vi "Scanning Motion One Direction for Y Multiple Readings per Point.vi"() -> ()   [LabVIEW 2021]
uses:
  <vilib>/Utility/file.llb/Write Delimited Spreadsheet (DBL).vi
  MID-main/Marlin Instrument Driver/Marlin Instrument Driver.lvlib
  <instrlib>/Siglent SDS 1000 2000 Series/Siglent SDS 1000 2000 Series.lvlib
panel:
  in  "Samples per pt":dbl=10.0
  in  "VISA resource name o-scope":refnum<visa-resource-name>="USB0::0xF4ED::0xEE3A::SDS1EDED5R2476::INSTR"
  in  "Measurement (0: Vpp)":u16(ring) items=["Vpp", "Vmax", "Vmin", "Vamp", "Vtop", "Vbase", "Vavg", "Mean", "Vrms", "Crms", "FOV", "FPRE", "ROV", "RPRE", "Period", "Freq", "+Wid", "-Wid", "Rise Time", "Fall Time", "Bwid", "+Duty", "-Duty"]
  in  "Source (1: Channel 1)":u16(ring)=1 items=["Channel 1"=1, "Channel 2"=2, "Channel 3"=3, "Channel 4"=4]
  in  "file path (dialog if empty)":path=path "C:/Users/scoughen/Documents/Printer Controll/Coughenour Programs/Scan Data/SimpleTransducer500kHzHighRes10SampleAvg0SecDelay7mmOffsetFromTransducerNewAmp.csv"
  in  "T":dbl
  in  "y Flag":string="Negative"
  in  "x Flag":string="Negative"
  in  "linearF":dbl=1000.0
  in  "E":dbl
  in  "rapidF":dbl=3000.0
  in  "zRes":dbl=0.5
  in  "yRes":dbl=1.0
  in  "xRes":dbl=0.5
  in  "zSize":dbl=80.0
  in  "ySize":dbl=10.0
  in  "xSize":dbl=50.0
  in  "zInit":dbl=155.0
  in  "yInit":dbl=168.0
  in  "xInit":dbl=115.0
  out "error out":errorcluster
  in  "error in (no error)":errorcluster
  in  "VISA resource name":refnum<visa-resource-name>="COM5"
  # "All Units in mm"
  # "Initial Position"
  # "Scan Size"
  # "Scan Resolution"
  # "Extrusion"
  # "Feed Rate"
  # "Read Delay (s)"
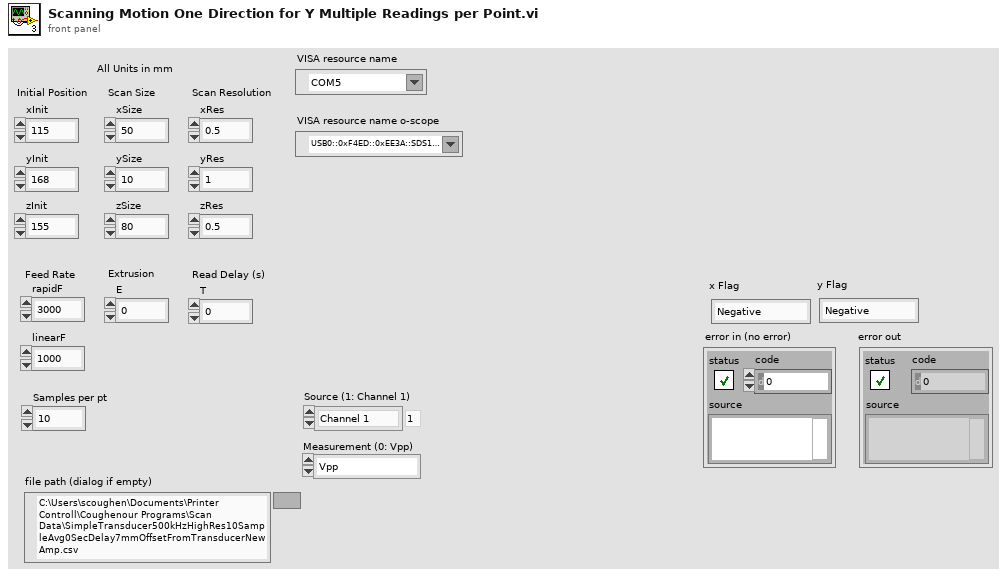
[diagram p1: front panel]
types:
  T1 = cluster{"E":dbl, "rapidF":dbl, "xInit":dbl, "yInit":dbl, "zInit":dbl}
  T2 = cluster{"E":dbl, "linearF":dbl, dbl, "yInit":dbl, "zInit":dbl}
  T3 = cluster{"E":dbl, "linearF":dbl, "xInit":dbl, dbl, "zInit":dbl}
  T4 = cluster{"E":dbl, "linearF":dbl, dbl, "zInit":dbl, "yInit":dbl}
  T5 = cluster{"E":dbl, "linearF":dbl, "xInit":dbl, "yInit":dbl, dbl}
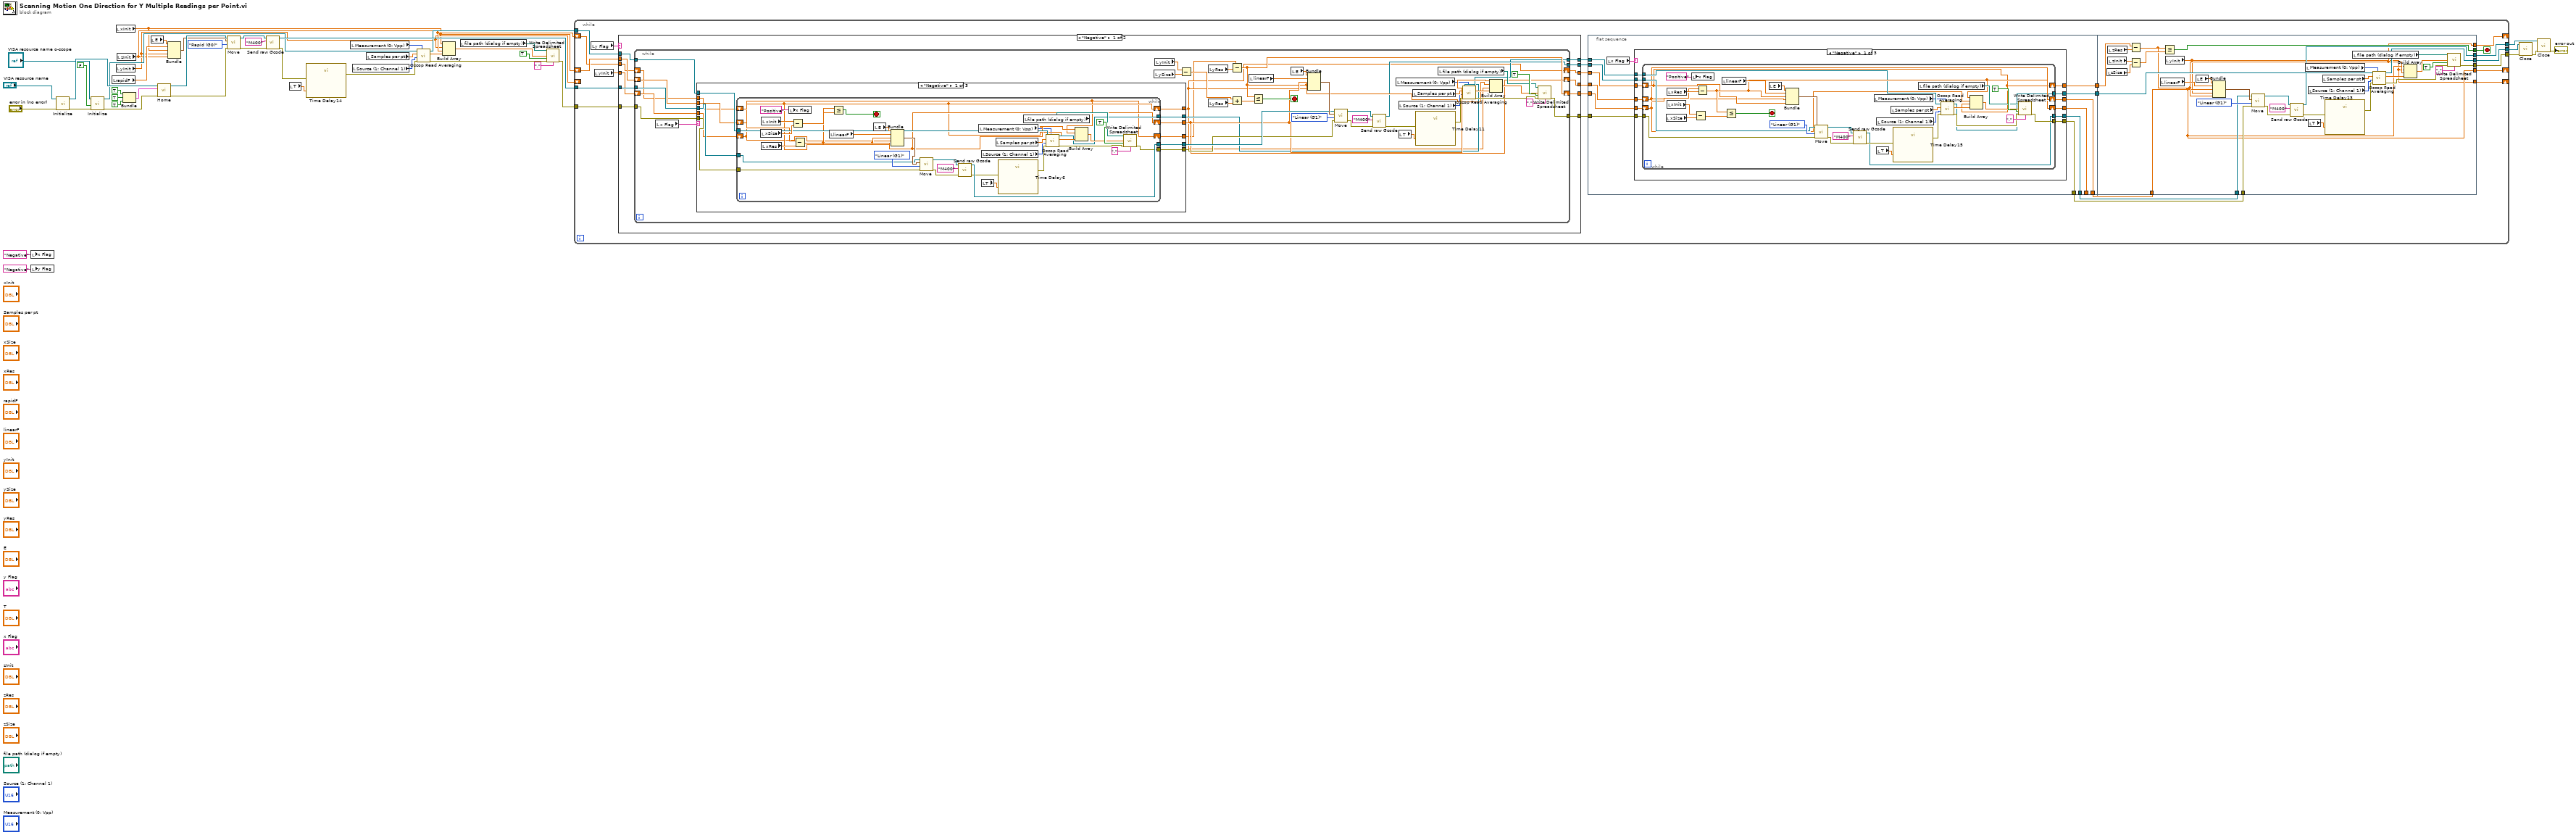
[diagram p0: block diagram]
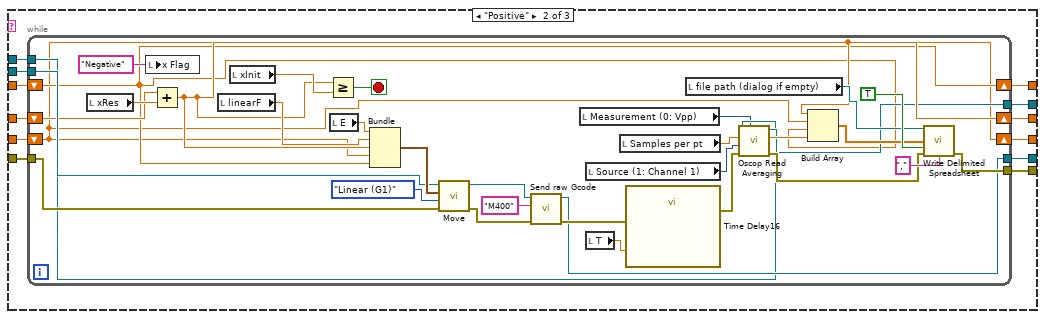
[diagram p2: hidden frame]
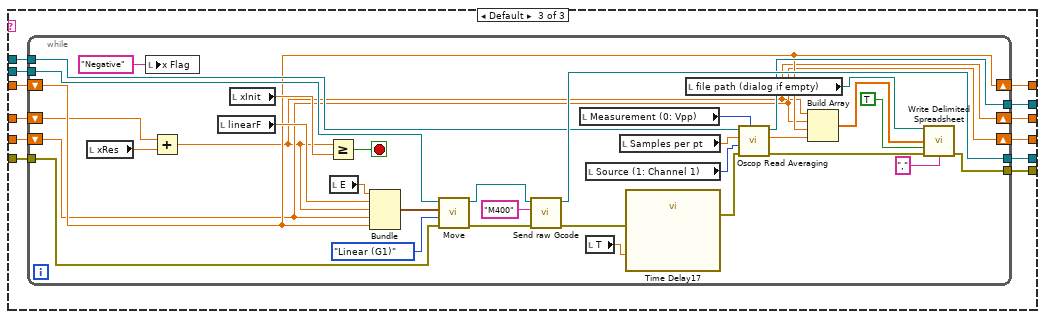
[diagram p3: hidden frame]
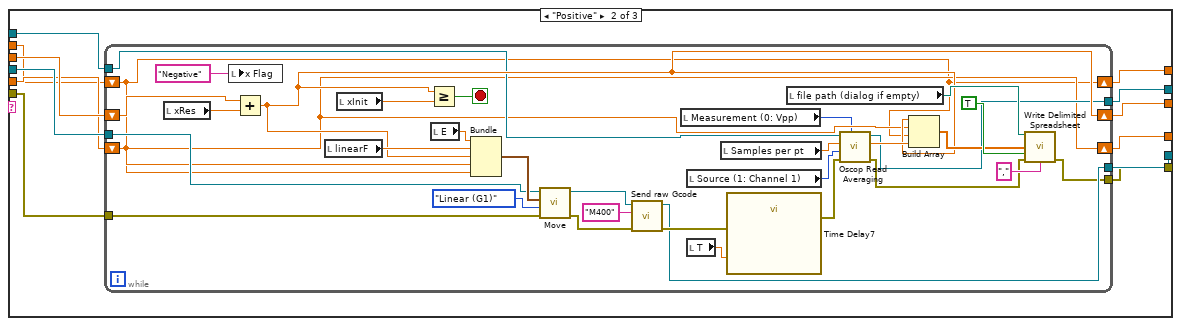
[diagram p4: hidden frame]
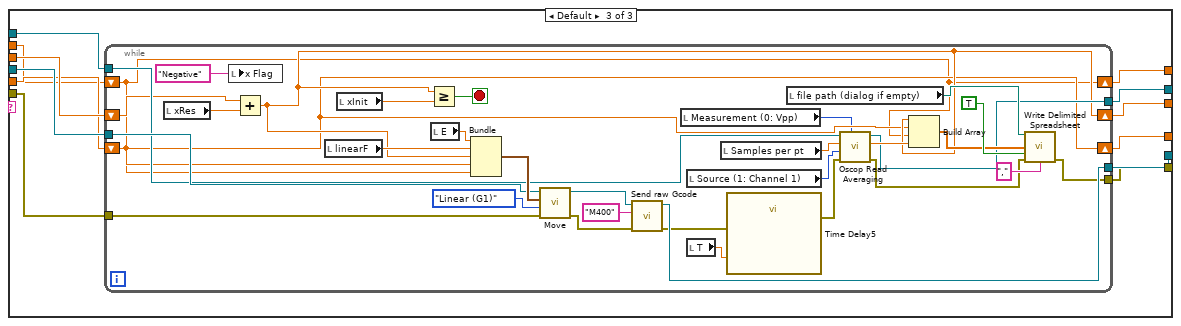
[diagram p5: hidden frame]
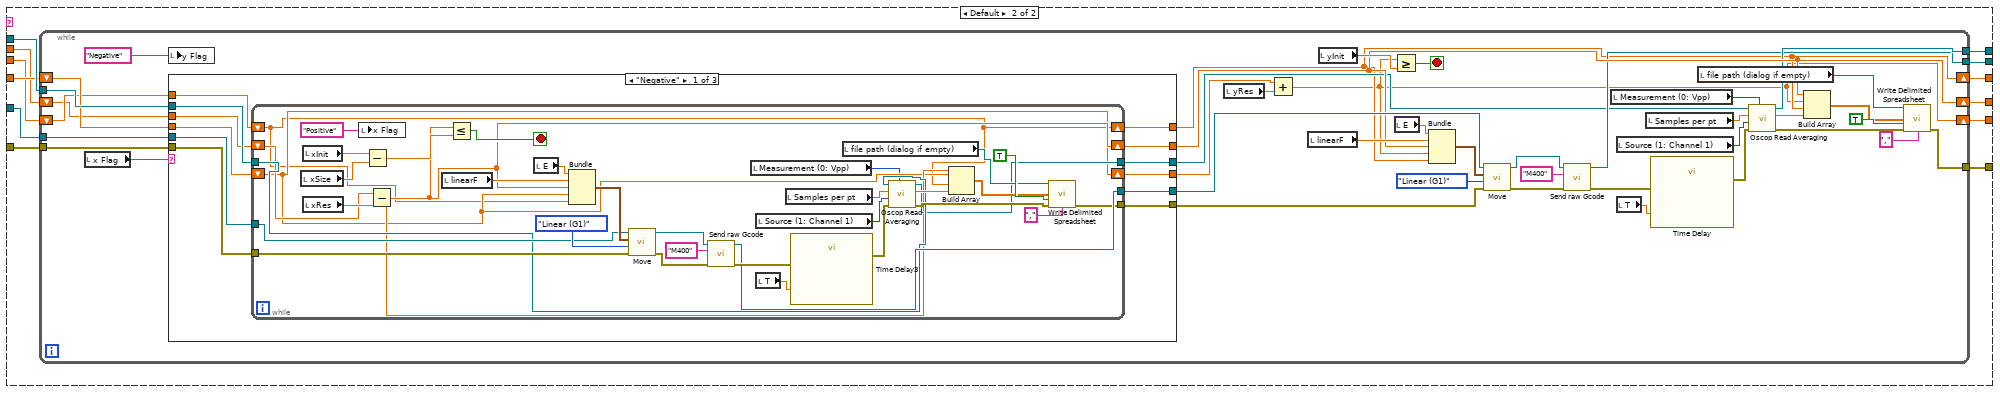
[diagram p6: hidden frame]
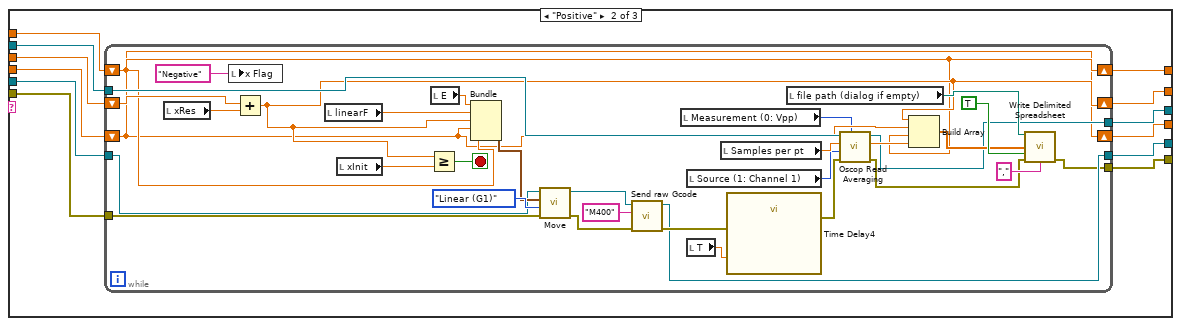
[diagram p7: hidden frame]
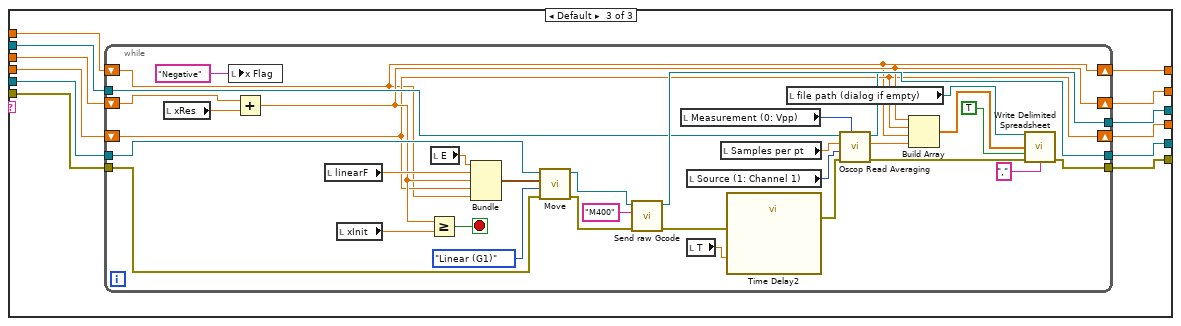
[diagram p8: hidden frame]
diagram:
  n1 = local write "x Flag"("Negative" ("x Flag")) -> ()
  n2 = local write "y Flag"("Negative" ("y Flag")) -> ()
  n3 = call <instrlib>:"Initialize.vi"("error in (no error)"="error in (no error)", "VISA resource name"="VISA resource name") -> ("error out"=w23:errorcluster, "VISA resource name out"=w43:refnum<visa-resource-name>)  [unwired: 8 in]
  n4 = call <instrlib>:"Initialize.vi"("error in (no error)"=w23, "Reset (True)"=FALSE, "VISA resource name"="VISA resource name o-scope") -> ("error out"=w22:errorcluster, "VISA resource name out"=w11:refnum<visa-resource-name>)  [unwired: 7 in]
  n5 = local read "rapidF"() -> (w33:dbl)
  n6 = local read "xInit"() -> (w6:dbl)
  n7 = local read "yInit"() -> (w7:dbl)
  n8 = local read "zInit"() -> (w8:dbl)
  n9 = Bundle(TRUE, TRUE, TRUE) -> (w39:cluster{bool, bool, bool})  [unwired: 1 in]
  n10 = local read "E"() -> (w32:dbl)
  n11 = call "Home.vi"("error in (no error)"=w22, "Axes"=w39, "VISA resource name"=w43) -> ("error out"=w38:errorcluster, "VISA resource name out"=w37:refnum<visa-resource-name>)  [unwired: 7 in]
  n12 = Bundle("E"=w32, "rapidF"=w33, "xInit"=w6, "yInit"=w7, "zInit"=w8) -> (w35:T1)  [unwired: 1 in]
  n13 = call "Move.vi"("error in (no error)"=w38, "type"=enum16{"Rapid (G0)", "Linear (G1)"}."Rapid (G0)" ("type 2"), "Distances"=w35, "VISA resource name"=w37) -> ("error out"=w27:errorcluster, "VISA resource name out"=w28:refnum<visa-resource-name>)  [unwired: 6 in]
  n14 = call "Send raw Gcode.vi"("error in (no error)"=w27, "Gcode"="M400", "VISA resource name"=w28) -> ("error out"=w25:errorcluster, "VISA resource name out"=w26:refnum<visa-resource-name>)  [unwired: 5 in, 2 out]
  n15 = local read "T"() -> (w29:dbl)
  n16 = call "Time Delay14"("error in (no error)"=w25, "Delay Time (s)"=w29) -> ("error out"=w13:errorcluster)  [unwired: 9 in]
  n17 = local read "Measurement (0: Vpp)"() -> (w9:u16)
  n18 = local read "Source (1: Channel 1)"() -> (w1:u16)
  n19 = local read "Samples per pt"() -> (w2:dbl)
  n20 = call "Oscop Read Averaging.vi"("Measurement (0: Vpp)"=w9, "error in (no error)"=w13, "Source (1: Channel 1)"=w1, "Numeric in"=w2, "VISA Refnum in"=w11) -> ("error out"=w14:errorcluster, "Numeric out"=w3:dbl, "VISA Refnum out"=w10:refnum<visa-resource-name>)  [unwired: 4 in]
  n21 = Build Array(w6, w7, w8, w3) -> (w15:dbl[])
  n22 = local read "file path (dialog if empty)"() -> (w5:path)
  n23 = call-poly <vilib>:"Write Delimited Spreadsheet.vi"("file path (dialog if empty)"=w5, "1D data"=w15, "append to file? (new file:F)"=TRUE, "error in (no error)"=w14, "delimiter (\\t)"="," ("delimiter (\\t)")) -> ("error out"=w12:errorcluster)  [unwired: 9 in, 1 out]
  n24 = while {
    tunnel: w26 -> [w71]
    tunnel: w12 -> [w70]
    tunnel: [w61] -> w34
    tunnel: [w60] -> w20
    tunnel: [w58] -> w18
    tunnel: w10 -> [w55]
    shift-right: [w50] -> _
    shift-left: w8 -> [w53]
    shift-right: [w49] -> _
    shift-left: w7 -> [_]
    shift-right: [w48] -> _
    shift-left: w6 -> [w54]
    stop <- w59 stop-if-true
    n25 = local read "y Flag"() -> (w69:string)
    n26 = local read "yInit"() -> (w47:dbl)
    n27 = case shown="\"Negative\"" w69 {
      tunnel: w71 -> [w267 w459]
      tunnel: [w264 w458] -> w68
      tunnel: w70 -> [w266 w457]
      tunnel: [w265 w456] -> w67
      tunnel: [w263 w455] -> w65
      tunnel: [w262 w454] -> w66
      tunnel: [w261 w453] -> w52
      tunnel: [w260 w452] -> w56
      tunnel: w55 -> [w259 w451]
      tunnel: w54 -> [w257 w448]
      tunnel: w47 -> [w258 w450]
      tunnel: w53 -> [w256 w449]
      frame "Negative" {
        n28 = while {
          tunnel: w267 -> [w308]
          tunnel: [w279] -> w264
          tunnel: w266 -> [w306]
          tunnel: [w282] -> w265
          tunnel: [w278] -> w260
          tunnel: w259 -> [w276]
          shift-right: [w280] -> w262
          shift-left: w258 -> [w273]
          shift-right: [w281] -> w263
          shift-left: w257 -> [w272]
          shift-right: [w275] -> w261
          shift-left: w256 -> [w271]
          stop <- w304 stop-if-true
          n29 = local read "x Flag"() -> (w303:string)
          n30 = case shown="\"Negative\"" w303 {
            tunnel: w308 -> [w322 w369 w414]
            tunnel: [w319 w368 w413] -> w307
            tunnel: w306 -> [w321 w367 w412]
            tunnel: [w320 w366 w410] -> w305
            tunnel: [w318 w365 w411] -> w281
            tunnel: [w317 w364 w409] -> w274
            tunnel: [w315 w363 w407] -> w277
            tunnel: w276 -> [w316 w362 w408]
            tunnel: w272 -> [w314 w361 w406]
            tunnel: w273 -> [w313 w360 w405]
            tunnel: w271 -> [w311 w359 w404]
            tunnel: [w312 w358 w403] -> w275
            frame "Negative" {
              n31 = while {
                tunnel: w322 -> [w355]
                tunnel: [w342] -> w319
                tunnel: w321 -> [w354]
                tunnel: [w332] -> w320
                tunnel: w316 -> [w331]
                tunnel: [w330] -> w315
                shift-right: [w328] -> w318
                shift-left: w314 -> [w329]
                shift-right: [w326] -> w317
                shift-left: w313 -> [w326]
                shift-right: [w327] -> w312
                shift-left: w311 -> [w327]
                stop <- w353 stop-if-true
                n32 = local read "xSize"() -> (w347:dbl)
                n33 = local read "xInit"() -> (w348:dbl)
                n34 = local read "xRes"() -> (w350:dbl)
                n35 = local write "x Flag"("Positive" ("x Flag")) -> ()
                n36 = Subtract(x=w348, y=w347) -> (x-y=w346:dbl)
                n37 = Subtract(x=w329, y=w350) -> (x-y=w328:dbl)
                n38 = local read "linearF"() -> (w351:dbl)
                n39 = Less Or Equal?(x=w328, y=w346) -> (x <= y?=w353:bool)
                n40 = local read "E"() -> (w352:dbl)
                n41 = Bundle("E"=w352, "linearF"=w351, w328, "yInit"=w326, "zInit"=w327) -> (w356:T2)  [unwired: 1 in]
                n42 = call "Move.vi"("error in (no error)"=w354, "type"=enum16{"Rapid (G0)", "Linear (G1)"}."Linear (G1)" ("type 2"), "Distances"=w356, "VISA resource name"=w355) -> ("error out"=w341:errorcluster, "VISA resource name out"=w343:refnum<visa-resource-name>)  [unwired: 6 in]
                n43 = call "Send raw Gcode.vi"("error in (no error)"=w341, "Gcode"="M400", "VISA resource name"=w343) -> ("error out"=w340:errorcluster, "VISA resource name out"=w342:refnum<visa-resource-name>)  [unwired: 5 in, 2 out]
                n44 = local read "Measurement (0: Vpp)"() -> (w325:u16)
                n45 = local read "Source (1: Channel 1)"() -> (w323:u16)
                n46 = local read "T"() -> (w345:dbl)
                n47 = local read "Samples per pt"() -> (w324:dbl)
                n48 = call "Time Delay6"("error in (no error)"=w340, "Delay Time (s)"=w345) -> ("error out"=w333:errorcluster)  [unwired: 9 in]
                n49 = local read "file path (dialog if empty)"() -> (w337:path)
                n50 = call "Oscop Read Averaging.vi"("Measurement (0: Vpp)"=w325, "error in (no error)"=w333, "Source (1: Channel 1)"=w323, "Numeric in"=w324, "VISA Refnum in"=w331) -> ("error out"=w334:errorcluster, "Numeric out"=w335:dbl, "VISA Refnum out"=w330:refnum<visa-resource-name>)  [unwired: 4 in]
                n51 = Build Array(w328, w326, w327, w335) -> (w336:dbl[])
                n52 = call-poly <vilib>:"Write Delimited Spreadsheet.vi"("file path (dialog if empty)"=w337, "1D data"=w336, "append to file? (new file:F)"=TRUE, "error in (no error)"=w334, "delimiter (\\t)"="," ("delimiter (\\t)")) -> ("error out"=w332:errorcluster)  [unwired: 9 in, 1 out]
              }
            }
            frame "Positive" {
              n53 = while {
                tunnel: w369 -> [w400]
                tunnel: [w387] -> w368
                tunnel: w367 -> [w399]
                tunnel: [w379] -> w366
                tunnel: [w377] -> w363
                tunnel: w362 -> [w376]
                shift-right: [w378] -> w365
                shift-left: w361 -> [w375]
                shift-right: [w374] -> w364
                shift-left: w360 -> [w374]
                shift-right: [w373] -> w358
                shift-left: w359 -> [w373]
                stop <- w398 stop-if-true
                n54 = local read "xRes"() -> (w396:dbl)
                n55 = local write "x Flag"("Negative" ("x Flag")) -> ()
                n56 = Add(x=w375, y=w396) -> (x+y=w378:dbl)
                n57 = local read "linearF"() -> (w395:dbl)
                n58 = local read "xInit"() -> (w397:dbl)
                n59 = Greater Or Equal?(x=w378, y=w397) -> (x >= y?=w398:bool)
                n60 = local read "E"() -> (w394:dbl)
                n61 = Bundle("E"=w394, "linearF"=w395, w378, "yInit"=w374, "zInit"=w373) -> (w401:T2)  [unwired: 1 in]
                n62 = call "Move.vi"("error in (no error)"=w399, "type"=enum16{"Rapid (G0)", "Linear (G1)"}."Linear (G1)" ("type 2"), "Distances"=w401, "VISA resource name"=w400) -> ("error out"=w390:errorcluster, "VISA resource name out"=w388:refnum<visa-resource-name>)  [unwired: 6 in]
                n63 = call "Send raw Gcode.vi"("error in (no error)"=w390, "Gcode"="M400", "VISA resource name"=w388) -> ("error out"=w389:errorcluster, "VISA resource name out"=w387:refnum<visa-resource-name>)  [unwired: 5 in, 2 out]
                n64 = local read "Measurement (0: Vpp)"() -> (w371:u16)
                n65 = local read "Source (1: Channel 1)"() -> (w370:u16)
                n66 = local read "T"() -> (w392:dbl)
                n67 = local read "Samples per pt"() -> (w372:dbl)
                n68 = call "Time Delay7"("error in (no error)"=w389, "Delay Time (s)"=w392) -> ("error out"=w380:errorcluster)  [unwired: 9 in]
                n69 = local read "file path (dialog if empty)"() -> (w384:path)
                n70 = call "Oscop Read Averaging.vi"("Measurement (0: Vpp)"=w371, "error in (no error)"=w380, "Source (1: Channel 1)"=w370, "Numeric in"=w372, "VISA Refnum in"=w376) -> ("error out"=w381:errorcluster, "Numeric out"=w382:dbl, "VISA Refnum out"=w377:refnum<visa-resource-name>)  [unwired: 4 in]
                n71 = Build Array(w378, w374, w373, w382) -> (w383:dbl[])
                n72 = call-poly <vilib>:"Write Delimited Spreadsheet.vi"("file path (dialog if empty)"=w384, "1D data"=w383, "append to file? (new file:F)"=TRUE, "error in (no error)"=w381, "delimiter (\\t)"="," ("delimiter (\\t)")) -> ("error out"=w379:errorcluster)  [unwired: 9 in, 1 out]
              }
            }
            frame Default {
              n73 = while {
                tunnel: w414 -> [w445]
                tunnel: [w434] -> w413
                tunnel: w412 -> [w444]
                tunnel: [w424] -> w410
                tunnel: w408 -> [w423]
                tunnel: [w422] -> w407
                shift-right: [w421] -> w411
                shift-left: w406 -> [w420]
                shift-right: [w419] -> w409
                shift-left: w405 -> [w419]
                shift-right: [w418] -> w403
                shift-left: w404 -> [w418]
                stop <- w443 stop-if-true
                n74 = local read "xRes"() -> (w441:dbl)
                n75 = local write "x Flag"("Negative" ("x Flag")) -> ()
                n76 = Add(x=w420, y=w441) -> (x+y=w421:dbl)
                n77 = local read "linearF"() -> (w440:dbl)
                n78 = local read "xInit"() -> (w442:dbl)
                n79 = Greater Or Equal?(x=w421, y=w442) -> (x >= y?=w443:bool)
                n80 = local read "E"() -> (w439:dbl)
                n81 = Bundle("E"=w439, "linearF"=w440, w421, "yInit"=w419, "zInit"=w418) -> (w446:T2)  [unwired: 1 in]
                n82 = call "Move.vi"("error in (no error)"=w444, "type"=enum16{"Rapid (G0)", "Linear (G1)"}."Linear (G1)" ("type 2"), "Distances"=w446, "VISA resource name"=w445) -> ("error out"=w433:errorcluster, "VISA resource name out"=w435:refnum<visa-resource-name>)  [unwired: 6 in]
                n83 = call "Send raw Gcode.vi"("error in (no error)"=w433, "Gcode"="M400", "VISA resource name"=w435) -> ("error out"=w432:errorcluster, "VISA resource name out"=w434:refnum<visa-resource-name>)  [unwired: 5 in, 2 out]
                n84 = local read "Measurement (0: Vpp)"() -> (w416:u16)
                n85 = local read "Source (1: Channel 1)"() -> (w415:u16)
                n86 = local read "T"() -> (w437:dbl)
                n87 = local read "Samples per pt"() -> (w417:dbl)
                n88 = call "Time Delay5"("error in (no error)"=w432, "Delay Time (s)"=w437) -> ("error out"=w425:errorcluster)  [unwired: 9 in]
                n89 = local read "file path (dialog if empty)"() -> (w429:path)
                n90 = call "Oscop Read Averaging.vi"("Measurement (0: Vpp)"=w416, "error in (no error)"=w425, "Source (1: Channel 1)"=w415, "Numeric in"=w417, "VISA Refnum in"=w423) -> ("error out"=w426:errorcluster, "Numeric out"=w427:dbl, "VISA Refnum out"=w422:refnum<visa-resource-name>)  [unwired: 4 in]
                n91 = Build Array(w421, w419, w418, w427) -> (w428:dbl[])
                n92 = call-poly <vilib>:"Write Delimited Spreadsheet.vi"("file path (dialog if empty)"=w429, "1D data"=w428, "append to file? (new file:F)"=TRUE, "error in (no error)"=w426, "delimiter (\\t)"="," ("delimiter (\\t)")) -> ("error out"=w424:errorcluster)  [unwired: 9 in, 1 out]
              }
            }
          }
          n93 = local read "ySize"() -> (w298:dbl)
          n94 = local read "yInit"() -> (w299:dbl)
          n95 = Subtract(x=w299, y=w298) -> (x-y=w294:dbl)
          n96 = local read "yRes"() -> (w300:dbl)
          n97 = local read "yRes"() -> (w295:dbl)
          n98 = Subtract(x=w274, y=w300) -> (x-y=w280:dbl)
          n99 = Add(x=w294, y=w295) -> (x+y=w296:dbl)
          n100 = local read "linearF"() -> (w301:dbl)
          n101 = Less Or Equal?(x=w280, y=w296) -> (x <= y?=w304:bool)
          n102 = local read "E"() -> (w302:dbl)
          n103 = Bundle("E"=w302, "linearF"=w301, "xInit"=w281, w280, "zInit"=w275) -> (w309:T3)  [unwired: 1 in]
          n104 = call "Move.vi"("error in (no error)"=w305, "type"=enum16{"Rapid (G0)", "Linear (G1)"}."Linear (G1)" ("type 2"), "Distances"=w309, "VISA resource name"=w307) -> ("error out"=w291:errorcluster, "VISA resource name out"=w292:refnum<visa-resource-name>)  [unwired: 6 in]
          n105 = call "Send raw Gcode.vi"("error in (no error)"=w291, "Gcode"="M400", "VISA resource name"=w292) -> ("error out"=w290:errorcluster, "VISA resource name out"=w279:refnum<visa-resource-name>)  [unwired: 5 in, 2 out]
          n106 = local read "Measurement (0: Vpp)"() -> (w270:u16)
          n107 = local read "Source (1: Channel 1)"() -> (w268:u16)
          n108 = local read "T"() -> (w297:dbl)
          n109 = local read "Samples per pt"() -> (w269:dbl)
          n110 = call "Time Delay11"("error in (no error)"=w290, "Delay Time (s)"=w297) -> ("error out"=w283:errorcluster)  [unwired: 9 in]
          n111 = local read "file path (dialog if empty)"() -> (w287:path)
          n112 = call "Oscop Read Averaging.vi"("Measurement (0: Vpp)"=w270, "error in (no error)"=w283, "Source (1: Channel 1)"=w268, "Numeric in"=w269, "VISA Refnum in"=w277) -> ("error out"=w284:errorcluster, "Numeric out"=w285:dbl, "VISA Refnum out"=w278:refnum<visa-resource-name>)  [unwired: 4 in]
          n113 = Build Array(w281, w280, w275, w285) -> (w286:dbl[])
          n114 = call-poly <vilib>:"Write Delimited Spreadsheet.vi"("file path (dialog if empty)"=w287, "1D data"=w286, "append to file? (new file:F)"=TRUE, "error in (no error)"=w284, "delimiter (\\t)"="," ("delimiter (\\t)")) -> ("error out"=w282:errorcluster)  [unwired: 9 in, 1 out]
        }
      }
      frame Default {
        n115 = while {
          tunnel: w459 -> [w497]
          tunnel: [w470] -> w458
          tunnel: w457 -> [w495]
          tunnel: [w473] -> w456
          tunnel: [w471] -> w452
          tunnel: w451 -> [w469]
          shift-right: [w467] -> w453
          shift-left: w450 -> [w466]
          shift-right: [w465] -> w454
          shift-left: w449 -> [w464]
          shift-right: [w472] -> w455
          shift-left: w448 -> [w463]
          stop <- w493 stop-if-true
          n116 = local read "x Flag"() -> (w492:string)
          n117 = local write "y Flag"("Negative" ("y Flag")) -> ()
          n118 = case shown="\"Negative\"" w492 {
            tunnel: w497 -> [w511 w558 w603]
            tunnel: [w508 w557 w602] -> w496
            tunnel: w495 -> [w510 w556 w601]
            tunnel: [w509 w555 w600] -> w494
            tunnel: [w507 w554 w599] -> w472
            tunnel: [w506 w553 w598] -> w485
            tunnel: [w504 w551 w597] -> w468
            tunnel: w469 -> [w505 w552 w596]
            tunnel: [w503 w550 w595] -> w467
            tunnel: w466 -> [w502 w547 w593]
            tunnel: w464 -> [w501 w548 w592]
            tunnel: w463 -> [w500 w549 w594]
            frame "Negative" {
              n119 = while {
                tunnel: w511 -> [w544]
                tunnel: [w529] -> w508
                tunnel: w510 -> [w543]
                tunnel: [w519] -> w509
                tunnel: w505 -> [w522]
                tunnel: [w521] -> w504
                shift-right: [w515] -> w503
                shift-left: w501 -> [w515]
                shift-right: [w518] -> w507
                shift-left: w500 -> [w517]
                shift-right: [w516] -> w506
                shift-left: w502 -> [w516]
                stop <- w542 stop-if-true
                n120 = local read "xSize"() -> (w536:dbl)
                n121 = local read "xInit"() -> (w535:dbl)
                n122 = local read "xRes"() -> (w539:dbl)
                n123 = local write "x Flag"("Positive" ("x Flag")) -> ()
                n124 = Subtract(x=w535, y=w536) -> (x-y=w534:dbl)
                n125 = Subtract(x=w517, y=w539) -> (x-y=w518:dbl)
                n126 = local read "linearF"() -> (w540:dbl)
                n127 = Less Or Equal?(x=w518, y=w534) -> (x <= y?=w542:bool)
                n128 = local read "E"() -> (w541:dbl)
                n129 = Bundle("E"=w541, "linearF"=w540, w518, "yInit"=w516, "zInit"=w515) -> (w545:T2)  [unwired: 1 in]
                n130 = call "Move.vi"("error in (no error)"=w543, "type"=enum16{"Rapid (G0)", "Linear (G1)"}."Linear (G1)" ("type 2"), "Distances"=w545, "VISA resource name"=w544) -> ("error out"=w532:errorcluster, "VISA resource name out"=w530:refnum<visa-resource-name>)  [unwired: 6 in]
                n131 = call "Send raw Gcode.vi"("error in (no error)"=w532, "Gcode"="M400", "VISA resource name"=w530) -> ("error out"=w531:errorcluster, "VISA resource name out"=w529:refnum<visa-resource-name>)  [unwired: 5 in, 2 out]
                n132 = local read "Measurement (0: Vpp)"() -> (w513:u16)
                n133 = local read "Source (1: Channel 1)"() -> (w512:u16)
                n134 = local read "T"() -> (w537:dbl)
                n135 = local read "Samples per pt"() -> (w514:dbl)
                n136 = call "Time Delay3"("error in (no error)"=w531, "Delay Time (s)"=w537) -> ("error out"=w520:errorcluster)  [unwired: 9 in]
                n137 = local read "file path (dialog if empty)"() -> (w526:path)
                n138 = call "Oscop Read Averaging.vi"("Measurement (0: Vpp)"=w513, "error in (no error)"=w520, "Source (1: Channel 1)"=w512, "Numeric in"=w514, "VISA Refnum in"=w522) -> ("error out"=w523:errorcluster, "Numeric out"=w524:dbl, "VISA Refnum out"=w521:refnum<visa-resource-name>)  [unwired: 4 in]
                n139 = Build Array(w518, w516, w515, w524) -> (w525:dbl[])
                n140 = call-poly <vilib>:"Write Delimited Spreadsheet.vi"("file path (dialog if empty)"=w526, "1D data"=w525, "append to file? (new file:F)"=TRUE, "error in (no error)"=w523, "delimiter (\\t)"="," ("delimiter (\\t)")) -> ("error out"=w519:errorcluster)  [unwired: 9 in, 1 out]
              }
            }
            frame "Positive" {
              n141 = while {
                tunnel: w558 -> [w589]
                tunnel: [w576] -> w557
                tunnel: w556 -> [w588]
                tunnel: [w569] -> w555
                tunnel: w552 -> [w567]
                tunnel: [w566] -> w551
                shift-right: [w565] -> w554
                shift-left: w549 -> [w564]
                shift-right: [w563] -> w550
                shift-left: w548 -> [w563]
                shift-right: [w562] -> w553
                shift-left: w547 -> [w562]
                stop <- w587 stop-if-true
                n142 = local read "xRes"() -> (w585:dbl)
                n143 = local write "x Flag"("Negative" ("x Flag")) -> ()
                n144 = Add(x=w564, y=w585) -> (x+y=w565:dbl)
                n145 = local read "linearF"() -> (w584:dbl)
                n146 = local read "xInit"() -> (w586:dbl)
                n147 = Greater Or Equal?(x=w565, y=w586) -> (x >= y?=w587:bool)
                n148 = local read "E"() -> (w583:dbl)
                n149 = Bundle("E"=w583, "linearF"=w584, w565, "yInit"=w562, "zInit"=w563) -> (w590:T2)  [unwired: 1 in]
                n150 = call "Move.vi"("error in (no error)"=w588, "type"=enum16{"Rapid (G0)", "Linear (G1)"}."Linear (G1)" ("type 2"), "Distances"=w590, "VISA resource name"=w589) -> ("error out"=w579:errorcluster, "VISA resource name out"=w577:refnum<visa-resource-name>)  [unwired: 6 in]
                n151 = call "Send raw Gcode.vi"("error in (no error)"=w579, "Gcode"="M400", "VISA resource name"=w577) -> ("error out"=w578:errorcluster, "VISA resource name out"=w576:refnum<visa-resource-name>)  [unwired: 5 in, 2 out]
                n152 = local read "Measurement (0: Vpp)"() -> (w561:u16)
                n153 = local read "Source (1: Channel 1)"() -> (w559:u16)
                n154 = local read "T"() -> (w581:dbl)
                n155 = local read "Samples per pt"() -> (w560:dbl)
                n156 = call "Time Delay4"("error in (no error)"=w578, "Delay Time (s)"=w581) -> ("error out"=w568:errorcluster)  [unwired: 9 in]
                n157 = local read "file path (dialog if empty)"() -> (w573:path)
                n158 = call "Oscop Read Averaging.vi"("Measurement (0: Vpp)"=w561, "error in (no error)"=w568, "Source (1: Channel 1)"=w559, "Numeric in"=w560, "VISA Refnum in"=w567) -> ("error out"=w570:errorcluster, "Numeric out"=w571:dbl, "VISA Refnum out"=w566:refnum<visa-resource-name>)  [unwired: 4 in]
                n159 = Build Array(w565, w562, w563, w571) -> (w572:dbl[])
                n160 = call-poly <vilib>:"Write Delimited Spreadsheet.vi"("file path (dialog if empty)"=w573, "1D data"=w572, "append to file? (new file:F)"=TRUE, "error in (no error)"=w570, "delimiter (\\t)"="," ("delimiter (\\t)")) -> ("error out"=w569:errorcluster)  [unwired: 9 in, 1 out]
              }
            }
            frame Default {
              n161 = while {
                tunnel: w603 -> [w634]
                tunnel: [w623] -> w602
                tunnel: w601 -> [w633]
                tunnel: [w613] -> w600
                tunnel: [w612] -> w597
                tunnel: w596 -> [w611]
                shift-right: [w610] -> w599
                shift-left: w594 -> [w609]
                shift-right: [w608] -> w598
                shift-left: w593 -> [w608]
                shift-right: [w607] -> w595
                shift-left: w592 -> [w607]
                stop <- w632 stop-if-true
                n162 = local read "xRes"() -> (w631:dbl)
                n163 = local write "x Flag"("Negative" ("x Flag")) -> ()
                n164 = Add(x=w609, y=w631) -> (x+y=w610:dbl)
                n165 = local read "linearF"() -> (w630:dbl)
                n166 = local read "xInit"() -> (w626:dbl)
                n167 = Greater Or Equal?(x=w610, y=w626) -> (x >= y?=w632:bool)
                n168 = local read "E"() -> (w629:dbl)
                n169 = Bundle("E"=w629, "linearF"=w630, w610, "yInit"=w608, "zInit"=w607) -> (w635:T2)  [unwired: 1 in]
                n170 = call "Move.vi"("error in (no error)"=w633, "type"=enum16{"Rapid (G0)", "Linear (G1)"}."Linear (G1)" ("type 2"), "Distances"=w635, "VISA resource name"=w634) -> ("error out"=w622:errorcluster, "VISA resource name out"=w624:refnum<visa-resource-name>)  [unwired: 6 in]
                n171 = call "Send raw Gcode.vi"("error in (no error)"=w622, "Gcode"="M400", "VISA resource name"=w624) -> ("error out"=w621:errorcluster, "VISA resource name out"=w623:refnum<visa-resource-name>)  [unwired: 5 in, 2 out]
                n172 = local read "Measurement (0: Vpp)"() -> (w605:u16)
                n173 = local read "Source (1: Channel 1)"() -> (w604:u16)
                n174 = local read "T"() -> (w627:dbl)
                n175 = local read "Samples per pt"() -> (w606:dbl)
                n176 = call "Time Delay2"("error in (no error)"=w621, "Delay Time (s)"=w627) -> ("error out"=w614:errorcluster)  [unwired: 9 in]
                n177 = local read "file path (dialog if empty)"() -> (w618:path)
                n178 = call "Oscop Read Averaging.vi"("Measurement (0: Vpp)"=w605, "error in (no error)"=w614, "Source (1: Channel 1)"=w604, "Numeric in"=w606, "VISA Refnum in"=w611) -> ("error out"=w615:errorcluster, "Numeric out"=w616:dbl, "VISA Refnum out"=w612:refnum<visa-resource-name>)  [unwired: 4 in]
                n179 = Build Array(w610, w608, w607, w616) -> (w617:dbl[])
                n180 = call-poly <vilib>:"Write Delimited Spreadsheet.vi"("file path (dialog if empty)"=w618, "1D data"=w617, "append to file? (new file:F)"=TRUE, "error in (no error)"=w615, "delimiter (\\t)"="," ("delimiter (\\t)")) -> ("error out"=w613:errorcluster)  [unwired: 9 in, 1 out]
              }
            }
          }
          n181 = local read "yRes"() -> (w489:dbl)
          n182 = Add(x=w485, y=w489) -> (x+y=w465:dbl)
          n183 = local read "linearF"() -> (w490:dbl)
          n184 = local read "yInit"() -> (w486:dbl)
          n185 = Greater Or Equal?(x=w465, y=w486) -> (x >= y?=w493:bool)
          n186 = local read "E"() -> (w491:dbl)
          n187 = Bundle("E"=w491, "linearF"=w490, "xInit"=w472, w465, "zInit"=w467) -> (w498:T3)  [unwired: 1 in]
          n188 = call "Move.vi"("error in (no error)"=w494, "type"=enum16{"Rapid (G0)", "Linear (G1)"}."Linear (G1)" ("type 2"), "Distances"=w498, "VISA resource name"=w496) -> ("error out"=w482:errorcluster, "VISA resource name out"=w483:refnum<visa-resource-name>)  [unwired: 6 in]
          n189 = call "Send raw Gcode.vi"("error in (no error)"=w482, "Gcode"="M400", "VISA resource name"=w483) -> ("error out"=w481:errorcluster, "VISA resource name out"=w470:refnum<visa-resource-name>)  [unwired: 5 in, 2 out]
          n190 = local read "Measurement (0: Vpp)"() -> (w462:u16)
          n191 = local read "Source (1: Channel 1)"() -> (w460:u16)
          n192 = local read "T"() -> (w487:dbl)
          n193 = local read "Samples per pt"() -> (w461:dbl)
          n194 = call "Time Delay"("error in (no error)"=w481, "Delay Time (s)"=w487) -> ("error out"=w475:errorcluster)  [unwired: 9 in]
          n195 = local read "file path (dialog if empty)"() -> (w478:path)
          n196 = call "Oscop Read Averaging.vi"("Measurement (0: Vpp)"=w462, "error in (no error)"=w475, "Source (1: Channel 1)"=w460, "Numeric in"=w461, "VISA Refnum in"=w468) -> ("error out"=w474:errorcluster, "Numeric out"=w476:dbl, "VISA Refnum out"=w471:refnum<visa-resource-name>)  [unwired: 4 in]
          n197 = Build Array(w472, w465, w467, w476) -> (w477:dbl[])
          n198 = call-poly <vilib>:"Write Delimited Spreadsheet.vi"("file path (dialog if empty)"=w478, "1D data"=w477, "append to file? (new file:F)"=TRUE, "error in (no error)"=w474, "delimiter (\\t)"="," ("delimiter (\\t)")) -> ("error out"=w473:errorcluster)  [unwired: 9 in, 1 out]
        }
      }
    }
    n199 = flat-sequence {
      tunnel: w68 -> [w83]
      tunnel: w67 -> [w82]
      tunnel: w52 -> [w81]
      tunnel: w66 -> [w80]
      tunnel: w65 -> [w79]
      tunnel: [w78] -> w62
      tunnel: [w77] -> w63
      tunnel: [w76] -> w64
      tunnel: [w75] -> _
      tunnel: [w74] -> w57
      tunnel: w56 -> [w73]
      tunnel: [w72] -> w51
      tunnel: w64 -> [w226]
      tunnel: w63 -> [w247]
      tunnel: w62 -> [w245]
      tunnel: [w231] -> w61
      tunnel: [w239] -> w60
      tunnel: [w240] -> w59
      tunnel: [w230] -> w58
      tunnel: w57 -> [w229]
      tunnel: w51 -> [w228]
      tunnel: [w227] -> w50
      tunnel: [w225] -> w49
      tunnel: [w226] -> w48
      frame #0 {
        n200 = local read "x Flag"() -> (w84:string)
        n201 = case shown="\"Negative\"" w84 {
          tunnel: w83 -> [w96 w143 w188]
          tunnel: [w93 w142 w187] -> w78
          tunnel: w82 -> [w95 w141 w186]
          tunnel: [w94 w140 w184] -> w77
          tunnel: [w92 w139 w185] -> w76
          tunnel: [w91 w138 w183] -> w75
          tunnel: w81 -> [w90 w137 w182]
          tunnel: w80 -> [w85 w136 w177]
          tunnel: w79 -> [w86 w135 w178]
          tunnel: [w89 w134 w181] -> w74
          tunnel: w73 -> [w88 w133 w180]
          tunnel: [w87 w132 w179] -> w72
          frame "Negative" {
            n202 = while {
              tunnel: w96 -> [w129]
              tunnel: [w105] -> w93
              tunnel: w95 -> [w128]
              tunnel: [w110] -> w94
              tunnel: [w104] -> w89
              tunnel: w88 -> [w103]
              shift-right: [w102] -> w87
              shift-left: w90 -> [w102]
              shift-right: [w100] -> w91
              shift-left: w85 -> [w100]
              shift-right: [w109] -> w92
              shift-left: w86 -> [w101]
              stop <- w127 stop-if-true
              n203 = local read "xSize"() -> (w121:dbl)
              n204 = local read "xRes"() -> (w124:dbl)
              n205 = local read "xInit"() -> (w122:dbl)
              n206 = local write "x Flag"("Positive" ("x Flag")) -> ()
              n207 = Subtract(x=w122, y=w121) -> (x-y=w120:dbl)
              n208 = Subtract(x=w101, y=w124) -> (x-y=w109:dbl)
              n209 = local read "linearF"() -> (w125:dbl)
              n210 = Less Or Equal?(x=w109, y=w120) -> (x <= y?=w127:bool)
              n211 = local read "E"() -> (w126:dbl)
              n212 = Bundle("E"=w126, "linearF"=w125, w109, "zInit"=w100, "yInit"=w102) -> (w130:T4)  [unwired: 1 in]
              n213 = call "Move.vi"("error in (no error)"=w128, "type"=enum16{"Rapid (G0)", "Linear (G1)"}."Linear (G1)" ("type 2"), "Distances"=w130, "VISA resource name"=w129) -> ("error out"=w117:errorcluster, "VISA resource name out"=w115:refnum<visa-resource-name>)  [unwired: 6 in]
              n214 = call "Send raw Gcode.vi"("error in (no error)"=w117, "Gcode"="M400", "VISA resource name"=w115) -> ("error out"=w116:errorcluster, "VISA resource name out"=w105:refnum<visa-resource-name>)  [unwired: 5 in, 2 out]
              n215 = local read "Measurement (0: Vpp)"() -> (w99:u16)
              n216 = local read "Source (1: Channel 1)"() -> (w97:u16)
              n217 = local read "T"() -> (w119:dbl)
              n218 = local read "Samples per pt"() -> (w98:dbl)
              n219 = call "Time Delay15"("error in (no error)"=w116, "Delay Time (s)"=w119) -> ("error out"=w108:errorcluster)  [unwired: 9 in]
              n220 = local read "file path (dialog if empty)"() -> (w112:path)
              n221 = call "Oscop Read Averaging.vi"("Measurement (0: Vpp)"=w99, "error in (no error)"=w108, "Source (1: Channel 1)"=w97, "Numeric in"=w98, "VISA Refnum in"=w103) -> ("error out"=w107:errorcluster, "Numeric out"=w106:dbl, "VISA Refnum out"=w104:refnum<visa-resource-name>)  [unwired: 4 in]
              n222 = Build Array(w109, w100, w102, w106) -> (w111:dbl[])
              n223 = call-poly <vilib>:"Write Delimited Spreadsheet.vi"("file path (dialog if empty)"=w112, "1D data"=w111, "append to file? (new file:F)"=TRUE, "error in (no error)"=w107, "delimiter (\\t)"="," ("delimiter (\\t)")) -> ("error out"=w110:errorcluster)  [unwired: 9 in, 1 out]
            }
          }
          frame "Positive" {
            n224 = while {
              tunnel: w143 -> [w174]
              tunnel: [w151] -> w142
              tunnel: w141 -> [w173]
              tunnel: [w156] -> w140
              tunnel: [w150] -> w134
              tunnel: w133 -> [w149]
              shift-right: [w148] -> w132
              shift-left: w137 -> [w148]
              shift-right: [w147] -> w138
              shift-left: w136 -> [w147]
              shift-right: [w155] -> w139
              shift-left: w135 -> [w165]
              stop <- w172 stop-if-true
              n225 = local read "xRes"() -> (w170:dbl)
              n226 = local write "x Flag"("Negative" ("x Flag")) -> ()
              n227 = Add(x=w165, y=w170) -> (x+y=w155:dbl)
              n228 = local read "linearF"() -> (w169:dbl)
              n229 = local read "xInit"() -> (w171:dbl)
              n230 = Greater Or Equal?(x=w155, y=w171) -> (x >= y?=w172:bool)
              n231 = local read "E"() -> (w168:dbl)
              n232 = Bundle("E"=w168, "linearF"=w169, w155, "zInit"=w147, "yInit"=w148) -> (w175:T4)  [unwired: 1 in]
              n233 = call "Move.vi"("error in (no error)"=w173, "type"=enum16{"Rapid (G0)", "Linear (G1)"}."Linear (G1)" ("type 2"), "Distances"=w175, "VISA resource name"=w174) -> ("error out"=w163:errorcluster, "VISA resource name out"=w161:refnum<visa-resource-name>)  [unwired: 6 in]
              n234 = call "Send raw Gcode.vi"("error in (no error)"=w163, "Gcode"="M400", "VISA resource name"=w161) -> ("error out"=w162:errorcluster, "VISA resource name out"=w151:refnum<visa-resource-name>)  [unwired: 5 in, 2 out]
              n235 = local read "Measurement (0: Vpp)"() -> (w146:u16)
              n236 = local read "Source (1: Channel 1)"() -> (w144:u16)
              n237 = local read "T"() -> (w166:dbl)
              n238 = local read "Samples per pt"() -> (w145:dbl)
              n239 = call "Time Delay16"("error in (no error)"=w162, "Delay Time (s)"=w166) -> ("error out"=w154:errorcluster)  [unwired: 9 in]
              n240 = local read "file path (dialog if empty)"() -> (w158:path)
              n241 = call "Oscop Read Averaging.vi"("Measurement (0: Vpp)"=w146, "error in (no error)"=w154, "Source (1: Channel 1)"=w144, "Numeric in"=w145, "VISA Refnum in"=w149) -> ("error out"=w153:errorcluster, "Numeric out"=w152:dbl, "VISA Refnum out"=w150:refnum<visa-resource-name>)  [unwired: 4 in]
              n242 = Build Array(w155, w147, w148, w152) -> (w157:dbl[])
              n243 = call-poly <vilib>:"Write Delimited Spreadsheet.vi"("file path (dialog if empty)"=w158, "1D data"=w157, "append to file? (new file:F)"=TRUE, "error in (no error)"=w153, "delimiter (\\t)"="," ("delimiter (\\t)")) -> ("error out"=w156:errorcluster)  [unwired: 9 in, 1 out]
            }
          }
          frame Default {
            n244 = while {
              tunnel: w188 -> [w219]
              tunnel: [w198] -> w187
              tunnel: w186 -> [w218]
              tunnel: [w202] -> w184
              tunnel: [w197] -> w181
              tunnel: w180 -> [w196]
              shift-right: [w192] -> w185
              shift-left: w178 -> [w194]
              shift-right: [w193] -> w183
              shift-left: w177 -> [w193]
              shift-right: [w195] -> w179
              shift-left: w182 -> [w195]
              stop <- w217 stop-if-true
              n245 = local read "xRes"() -> (w215:dbl)
              n246 = local write "x Flag"("Negative" ("x Flag")) -> ()
              n247 = Add(x=w194, y=w215) -> (x+y=w192:dbl)
              n248 = local read "linearF"() -> (w214:dbl)
              n249 = local read "xInit"() -> (w216:dbl)
              n250 = Greater Or Equal?(x=w192, y=w216) -> (x >= y?=w217:bool)
              n251 = local read "E"() -> (w213:dbl)
              n252 = Bundle("E"=w213, "linearF"=w214, w192, "zInit"=w193, "yInit"=w195) -> (w220:T4)  [unwired: 1 in]
              n253 = call "Move.vi"("error in (no error)"=w218, "type"=enum16{"Rapid (G0)", "Linear (G1)"}."Linear (G1)" ("type 2"), "Distances"=w220, "VISA resource name"=w219) -> ("error out"=w208:errorcluster, "VISA resource name out"=w209:refnum<visa-resource-name>)  [unwired: 6 in]
              n254 = call "Send raw Gcode.vi"("error in (no error)"=w208, "Gcode"="M400", "VISA resource name"=w209) -> ("error out"=w207:errorcluster, "VISA resource name out"=w198:refnum<visa-resource-name>)  [unwired: 5 in, 2 out]
              n255 = local read "Measurement (0: Vpp)"() -> (w191:u16)
              n256 = local read "Source (1: Channel 1)"() -> (w189:u16)
              n257 = local read "T"() -> (w211:dbl)
              n258 = local read "Samples per pt"() -> (w190:dbl)
              n259 = call "Time Delay17"("error in (no error)"=w207, "Delay Time (s)"=w211) -> ("error out"=w200:errorcluster)  [unwired: 9 in]
              n260 = local read "file path (dialog if empty)"() -> (w204:path)
              n261 = call "Oscop Read Averaging.vi"("Measurement (0: Vpp)"=w191, "error in (no error)"=w200, "Source (1: Channel 1)"=w189, "Numeric in"=w190, "VISA Refnum in"=w196) -> ("error out"=w199:errorcluster, "Numeric out"=w201:dbl, "VISA Refnum out"=w197:refnum<visa-resource-name>)  [unwired: 4 in]
              n262 = Build Array(w192, w193, w195, w201) -> (w203:dbl[])
              n263 = call-poly <vilib>:"Write Delimited Spreadsheet.vi"("file path (dialog if empty)"=w204, "1D data"=w203, "append to file? (new file:F)"=TRUE, "error in (no error)"=w199, "delimiter (\\t)"="," ("delimiter (\\t)")) -> ("error out"=w202:errorcluster)  [unwired: 9 in, 1 out]
            }
          }
        }
      }
      frame #1 {
        n264 = local read "zSize"() -> (w243:dbl)
        n265 = local read "zRes"() -> (w241:dbl)
        n266 = local read "zInit"() -> (w242:dbl)
        n267 = Subtract(x=w228, y=w241) -> (x-y=w227:dbl)
        n268 = Subtract(x=w242, y=w243) -> (x-y=w244:dbl)
        n269 = local read "linearF"() -> (w250:dbl)
        n270 = Less Or Equal?(x=w227, y=w244) -> (x <= y?=w240:bool)
        n271 = local read "yInit"() -> (w225:dbl)
        n272 = local read "E"() -> (w251:dbl)
        n273 = Bundle("E"=w251, "linearF"=w250, "xInit"=w226, "yInit"=w225, w227) -> (w249:T5)  [unwired: 1 in]
        n274 = call "Move.vi"("error in (no error)"=w247, "type"=enum16{"Rapid (G0)", "Linear (G1)"}."Linear (G1)" ("type 2"), "Distances"=w249, "VISA resource name"=w245) -> ("error out"=w254:errorcluster, "VISA resource name out"=w253:refnum<visa-resource-name>)  [unwired: 6 in]
        n275 = call "Send raw Gcode.vi"("error in (no error)"=w254, "Gcode"="M400", "VISA resource name"=w253) -> ("error out"=w255:errorcluster, "VISA resource name out"=w231:refnum<visa-resource-name>)  [unwired: 5 in, 2 out]
        n276 = local read "Measurement (0: Vpp)"() -> (w224:u16)
        n277 = local read "Source (1: Channel 1)"() -> (w222:u16)
        n278 = local read "T"() -> (w252:dbl)
        n279 = local read "Samples per pt"() -> (w223:dbl)
        n280 = call "Time Delay13"("error in (no error)"=w255, "Delay Time (s)"=w252) -> ("error out"=w234:errorcluster)  [unwired: 9 in]
        n281 = local read "file path (dialog if empty)"() -> (w235:path)
        n282 = call "Oscop Read Averaging.vi"("Measurement (0: Vpp)"=w224, "error in (no error)"=w234, "Source (1: Channel 1)"=w222, "Numeric in"=w223, "VISA Refnum in"=w229) -> ("error out"=w233:errorcluster, "Numeric out"=w232:dbl, "VISA Refnum out"=w230:refnum<visa-resource-name>)  [unwired: 4 in]
        n283 = Build Array(w226, w225, w227, w232) -> (w236:dbl[])
        n284 = call-poly <vilib>:"Write Delimited Spreadsheet.vi"("file path (dialog if empty)"=w235, "1D data"=w236, "append to file? (new file:F)"=TRUE, "error in (no error)"=w233, "delimiter (\\t)"="," ("delimiter (\\t)")) -> ("error out"=w239:errorcluster)  [unwired: 9 in, 1 out]
      }
    }
  }
  n285 = call "Close.vi"("error in (no error)"=w20, "VISA resource name"=w18) -> ("error out"=w19:errorcluster)  [unwired: 9 in]
  n286 = call "Close.vi"("error in (no error)"=w19, "VISA resource name"=w34) -> ("error out"=→"error out":errorcluster)  [unwired: 9 in]
